vi "Get Data Logging Session Specification.vi"(8 "error in (no error)":errorcluster, 10 "Session Name in":string, 11 "Data Logging Manager Ref in":T2) -> (0 "error out":errorcluster, 1 "Data Logging Specification Ref out":T1, 2 "Session Name out":string, 3 "Data Logging Manager Ref out":T2)   [LabVIEW 2020, in "NI_VS Data Logging API.lvlib"]
doc: "Gets the reference to the data logging specification specified by <B>Session Name in</B>."
uses:
  <vilib>/NI VeriStand/Execution/DataLogging/NI_VS Data Logging API.lvlib
  <vilib>/NI VeriStand/Execution/DataLogging/IDataLogging Ref.ctl
  NationalInstruments.VeriStand.ClientAPI
  <vilib>/NI VeriStand/Execution/DataLogging/DataLoggingSpecification Ref.ctl
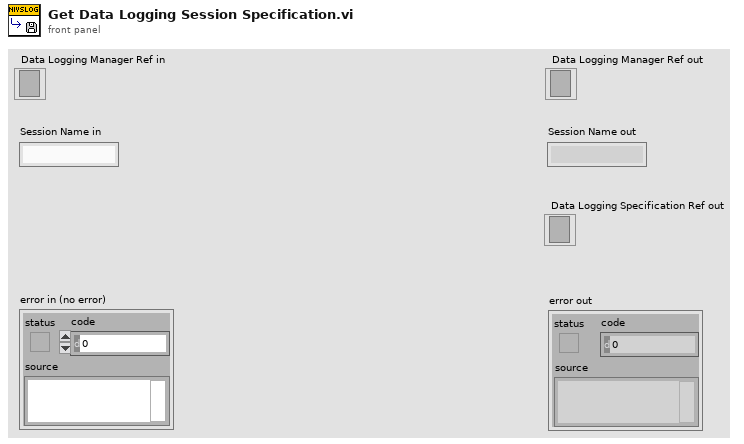
[diagram p1: front panel]
types:
  T1 = typedef "NI_VS Data Logging API.lvlib/DataLoggingSpecification Ref.ctl" = refnum<k24>
  T2 = typedef "NI_VS Data Logging API.lvlib/IDataLogging Ref.ctl" = refnum<k24>
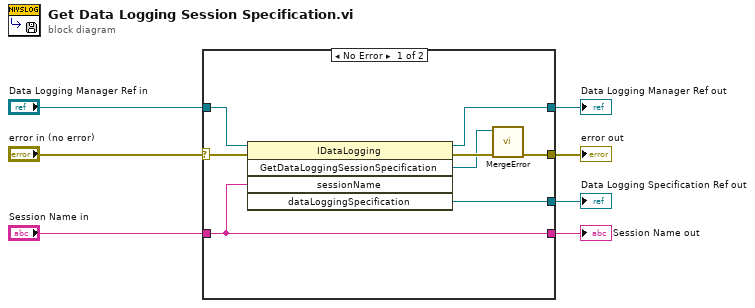
[diagram p0: block diagram]
diagram:
  n1 = case shown="No Error" "error in (no error)" {
    selector: "error in (no error)" -> [w13 w18]
    tunnel: [w10 w18] -> w6
    tunnel: [w9 w17] -> w5
    tunnel: "Data Logging Manager Ref in" -> [w15 w17]
    tunnel: [w14 w16] -> w3
    tunnel: "Session Name in" -> [w14 w16]
    tunnel: [w8 _] -> w1
    frame No Error {
      n2 = invoke class="IDataLogging" method="GetDataLoggingSessionSpecification"(reference=w15, error in=w13, "sessionName"=w14) -> (reference out=w9:T2, error out=w12:errorcluster, "GetDataLoggingSessionSpecification"=w11:refnum<k24>, "dataLoggingSpecification"=w8:refnum<k24>)  [unwired: 2 in, 1 out]
      n3 = call <vilib>:"MergeError.vi"("error in (no error)"=w12, "Error"=w11) -> ("error out"=w10:errorcluster)  [unwired: 9 out]
    }
    frame Error {
    }
  }
  "Data Logging Manager Ref out" <- w5
  "error out" <- w6
  "Session Name out" <- w3
  "Data Logging Specification Ref out" <- w1
